vi "SPD.Update Meas Grid control.vi"(6 "Meas.Grid Setup":refnum<vi>, 8 "error in (no error)":errorcluster, 11 "SPD.Stand Ctrl in":T1 {"spdDeviceSession"."hidSPD.Sturtup Values"."HV_bias" format="%#_6p, V"; "spdDeviceSession"."hidSPD.Sturtup Values"."TSet" format="%#_6p, DegC"; "spdDeviceSession"."hidSPD.Controller"."HV_bias" format="%#_6p, V"; "spdDeviceSession"."hidSPD.Controller"."TSet" format="%#_6p, DegC"}) -> (0 "error out":errorcluster, 3 "SPD.Stand Ctrl out":T1 {"spdDeviceSession"."hidSPD.Sturtup Values"."HV_bias" format="%#_6p, V"; "spdDeviceSession"."hidSPD.Sturtup Values"."TSet" format="%#_6p, DegC"; "spdDeviceSession"."hidSPD.Controller"."HV_bias" format="%#_6p, V"; "spdDeviceSession"."hidSPD.Controller"."TSet" format="%#_6p, DegC"})   [LabVIEW 2018]
uses:
  SPD Measurements/typedefs/SPD.Grid Meas Setup.ctl
  SPD Measurements/typedefs/SPD.Test Range.ctl
  typedefs/SPD.Stand Ctrl.ctl
  Instruments/SPD HID Interface/hidSPDLibForLabView/LibVIs/hidSPD Controls/hidSPD Device Session.ctl
  Instruments/SPD HID Interface/hidSPDLibForLabView/LibVIs/hidSPD Controls/hidSPD.SPD specification.ctl
  Instruments/SPD HID Interface/hidSPDLibForLabView/LibVIs/hidSPD Controls/hidSPD SPD Diod Case.ctl
  Instruments/SPD HID Interface/hidSPDLibForLabView/LibVIs/hidSPD Controls/hidSPD SPD Type.ctl
  Instruments/SPD HID Interface/hidSPDLibForLabView/LibVIs/hidSPD Controls/hidSPD.STB Frequency.ctl
  Instruments/SPD HID Interface/hidSPDLibForLabView/LibVIs/hidSPD Controls/hidSPD Controller.ctl
  Instruments/KC705 DevBoard/typedefs/DevB.Session.ctl
  Instruments/KeySight 53230A/typedefs/FreqC.Session.ctl
  Instruments/KeySight 8164B/KeySight 8164B LAN InstrLib/typedefs/KeySight 8164B control.ctl
  Instruments/LeCroy SDA830/typedefs/LeCroy.Session.ctl
  typedefs/SPD.Events.ctl
  ConfigFile/SPD.Config File ctrl.ctl
  <vilib>/Utility/config.llb/Config Data RefNum.ctl
  typedefs/SPD.Meas Grid.ctl
  typedefs/SPD.Queues.ctl
  typedefs/SPD.Stand state.ctl
  Instruments/SPD HID Interface/hidSPDLibForLabView/hidSPDLibForLabView.lvlib
  Instruments/KeySight 8164B/KeySight 8164B LAN InstrLib.lvlib
  <vilib>/Utility/config.llb/NI_LVConfig.lvlib
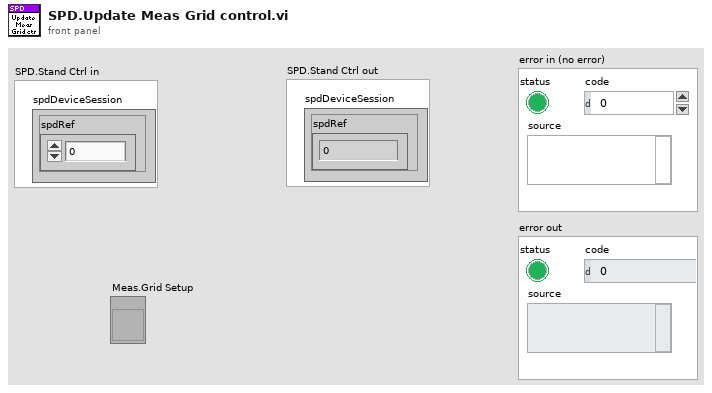
[diagram p1: front panel]
types:
  T1 = typedef "SPD.Stand Ctrl.ctl" = cluster{"spdDeviceSession":T2, "DevBSession":T8, "FreqCSession":T9, "8164BSession":T10, "LeCroySession":T11, "Events":T12, "configFile":T13, "SPD.Meas Grid":T15, "SPD.Queues":T16, "Console":refnum<vi>}
  T2 = typedef "hidSPDLibForLabView.lvlib/hidSPD Device Session.ctl" = cluster{"spdRef":u64, "connected":bool, "spdName":string, "specification":T3, "hidSPD.Controller":T7, "hidSPD.Sturtup Values":T7}
  T3 = typedef "hidSPDLibForLabView.lvlib/hidSPD.SPD specification.ctl" = cluster{"diod case":T4, "type":T5, "frequency":T6}
  T4 = typedef "hidSPDLibForLabView.lvlib/hidSPD SPD Diod Case.ctl" = enum16{"Unknown", "default", "butterfly"}
  T5 = typedef "hidSPDLibForLabView.lvlib/hidSPD SPD Type.ctl" = enum16{"Unknown", "Free Run", "Gate"}
  T6 = typedef "hidSPDLibForLabView.lvlib/hidSPD.STB Frequency.ctl" = enum16{"Unknown", "312", "1250"}
  T7 = typedef "hidSPDLibForLabView.lvlib/hidSPD Controller.ctl" = cluster{"TSet":sgl, "HV_bias":sgl, "DDS_stb_code":u16}
  T8 = typedef "DevB.Session.ctl" = cluster{"DevBRef":refnum<visa-resource-name>, "connected":bool}
  T9 = typedef "FreqC.Session.ctl" = cluster{"FreqCRef":refnum<visa-resource-name>, "timeout":dbl, "Gate":dbl, "connected":bool}
  T10 = typedef "KeySight 8164B LAN InstrLib.lvlib/KeySight 8164B control.ctl" = cluster{"Connection ID":refnum<k5>, "Connected":bool, "Info":string, "Slots Info":string[]}
  T11 = typedef "LeCroy.Session.ctl" = cluster{"LeCroySession":refnum<visa-resource-name>, "connected":bool}
  T12 = typedef "SPD.Events.ctl" = cluster{"DCRTest":refnum<user-event>, "Stop":refnum<user-event>}
  T13 = typedef "SPD.Config File ctrl.ctl" = cluster{"configFile ref":T14, "configFile path":path, "equipmentFile ref":T14}
  T14 = typedef "NI_LVConfig.lvlib/Config Data RefNum.ctl" = refnum<k1>
  T15 = typedef "SPD.Meas Grid.ctl" = cluster{"DateTime":string, "DT":dbl[], "Insensitivity":dbl[], "Temprature":dbl[], "Stb_code":dbl[], "HV_Bias":dbl[][][][]}
  T16 = typedef "SPD.Queues.ctl" = cluster{"state queue":refnum<queue>}
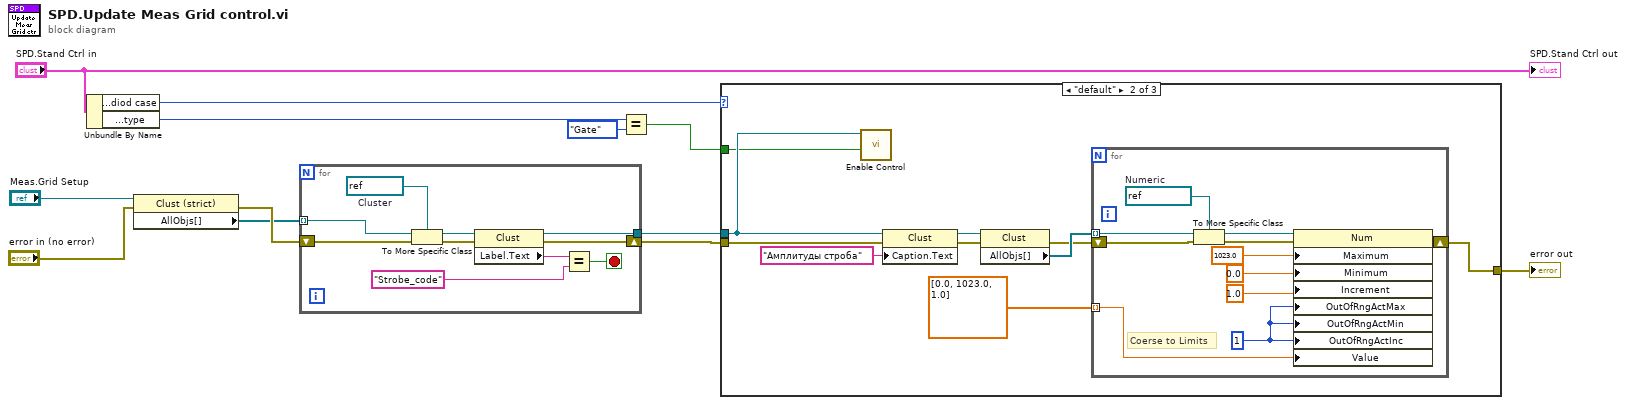
[diagram p0: block diagram]
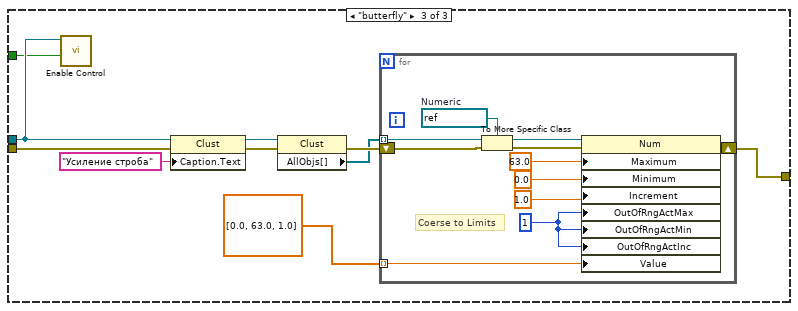
[diagram p3: hidden frame]
diagram:
  n1 = Unbundle By Name("SPD.Stand Ctrl in") -> ("spdDeviceSession.specification.diod case"=w6:T4, "spdDeviceSession.specification.type"=w3:T5)
  n2 = property class="Clust (strict)"(reference="Meas.Grid Setup", error in="error in (no error)") -> (error out=w12:errorcluster, "AllObjs[]"=w4:refnum<vi>[])  [unwired: 1 out]
  n3 = for {
    tunnel: [w13] -> w5
    shift-right: [w19] -> w7
    shift-left: w12 -> [w20]
    tunnel: w4 -> [w15] mode=indexing
    stop <- w14 stop-if-true
    w21 = refnum<vi> refnum  # Cluster
    n4 = To More Specific Class(target class=w21, reference=w15, error in=w20) -> (specific class reference=w18:refnum<vi>, error out=w19:errorcluster)
    n5 = property class="Clust"(reference=w18) -> (reference out=w13:refnum<vi>, "Label.Text"=w17:string)  [unwired: 1 in, 1 out]
    n6 = Equal?(x=w17, y="Strobe_code" ("x")) -> (x = y?=w14:bool)
  }
  n7 = Equal?(x=w3, y=hidSPD_SPD_Type."Gate") -> (x = y?=w1:bool)
  n8 = case shown="\"default\"" w6 {
    tunnel: [w22 w32 w53] -> w9
    tunnel: w5 -> [_ w31 w52]
    tunnel: w7 -> [w22 w30 w51]
    tunnel: w1 -> [_ w24 w45]
    frame "Unknown" {
    }
    frame "default" {
      n9 = call "Enable Control.vi"("enable"=w24, "Control"=w31) -> ()  [unwired: 10 in]
      n10 = property class="Clust"(reference=w31, error in=w30, "Caption.Text"="Амплитуды строба") -> (reference out=w27:refnum<vi>, error out=w28:errorcluster)
      n11 = property class="Clust"(reference=w27, error in=w28) -> (error out=w25:errorcluster, "AllObjs[]"=w26:refnum<vi>[])  [unwired: 1 out]
      n12 = for {
        tunnel: w26 -> [w43] mode=indexing
        shift-right: [w39] -> w32
        shift-left: w25 -> [w40]
        tunnel: dbl[] [0.0, 1023.0, 1.0] ("Data Entry Limits:Maximum") -> [w33] mode=indexing
        w34 = u8 1 ("Response to Value Outside Limits:Maximum")
        w42 = refnum<vi> refnum  # Numeric
        # "Coerse to Limits"
        n13 = To More Specific Class(target class=w42, reference=w43, error in=w40) -> (specific class reference=w41:refnum<vi>, error out=w38:errorcluster)
        n14 = property class="Num"(reference=w41, error in=w38, "Maximum"=1023.0 ("Data Entry Limits:Maximum"), "Minimum"=0.0 ("Data Entry Limits:Minimum"), "Increment"=1.0 ("Data Entry Limits:Increment"), "OutOfRngActMax"=w34, "OutOfRngActMin"=w34, "OutOfRngActInc"=w34, "Value"=w33) -> (error out=w39:errorcluster)  [unwired: 1 out]
      }
    }
    frame "butterfly" {
      n15 = call "Enable Control.vi"("enable"=w45, "Control"=w52) -> ()  [unwired: 10 in]
      n16 = property class="Clust"(reference=w52, error in=w51, "Caption.Text"="Усиление строба") -> (reference out=w49:refnum<vi>, error out=w48:errorcluster)
      n17 = property class="Clust"(reference=w49, error in=w48) -> (error out=w47:errorcluster, "AllObjs[]"=w46:refnum<vi>[])  [unwired: 1 out]
      n18 = for {
        tunnel: w46 -> [w64] mode=indexing
        shift-right: [w60] -> w53
        shift-left: w47 -> [w61]
        tunnel: dbl[] [0.0, 63.0, 1.0] ("Data Entry Limits:Maximum") -> [w54] mode=indexing
        w55 = u8 1 ("Response to Value Outside Limits:Maximum")
        w63 = refnum<vi> refnum  # Numeric
        # "Coerse to Limits"
        n19 = To More Specific Class(target class=w63, reference=w64, error in=w61) -> (specific class reference=w62:refnum<vi>, error out=w59:errorcluster)
        n20 = property class="Num"(reference=w62, error in=w59, "Maximum"=63.0 ("Data Entry Limits:Maximum"), "Minimum"=0.0 ("Data Entry Limits:Minimum"), "Increment"=1.0 ("Data Entry Limits:Increment"), "OutOfRngActMax"=w55, "OutOfRngActMin"=w55, "OutOfRngActInc"=w55, "Value"=w54) -> (error out=w60:errorcluster)  [unwired: 1 out]
      }
    }
  }
  "error out" <- w9
  "SPD.Stand Ctrl out" <- "SPD.Stand Ctrl in"
